vi "Check Chip Selection.vi"(6 "chip select":enum16{"1st chip", "2nd chip"}(ring), 8 "error in (no error)":errorcluster, 11 "cluster of private data in":T1={"FPGA VI Reference"=refnum, "device index"=0, "screen size"=enum."8x1", "font size"=enum."5x8", "auto wrap"=FALSE, "alignment"=enum."None", "number of line"=enum."2 lines", "shift 0"=0, "entry mode 0"=enum."increment & no shift", "shift 1"=0, "entry mode 1"=enum."increment & no shift"}) -> (0 "error out":errorcluster, 3 "cluster of private data out":T1={"FPGA VI Reference"=refnum, "device index"=0, "screen size"=enum."8x1", "font size"=enum."5x8", "auto wrap"=FALSE, "alignment"=enum."None", "number of line"=enum."2 lines", "shift 0"=0, "entry mode 0"=enum."increment & no shift", "shift 1"=0, "entry mode 1"=enum."increment & no shift"})   [LabVIEW 2017, in "HD44780.lvclass"]
uses:
  HD44780.lvclass
  Common/HD44780 Common.lvlib
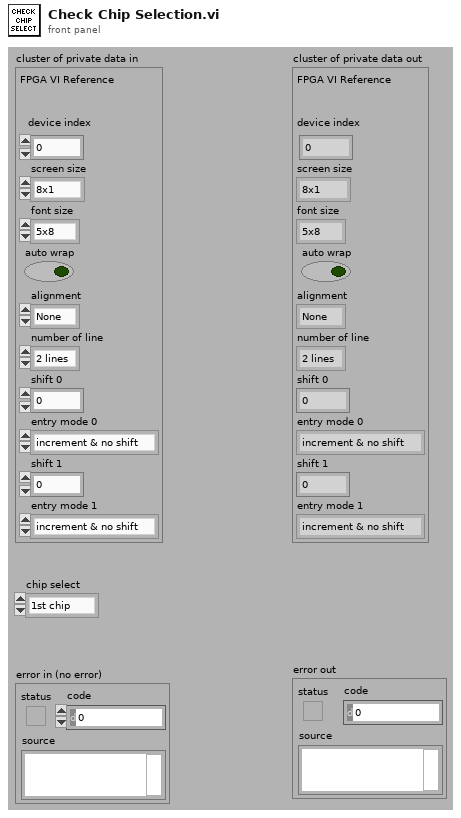
[diagram p1: front panel]
types:
  T1 = cluster{"FPGA VI Reference":refnum<k20>, "device index":i8, "screen size":enum8{"8x1", "8x2", "12x4", "16x1", "16x2", "16x4", "20x1", "20x2", "20x4", "24x1", "24x2", "40x2", "40x4"}, "font size":enum8{"5x8", "5x10"}, "auto wrap":bool, "alignment":enum16{"None", "Left", "Center", "Right"}, "number of line":enum8{"1 line", "2 lines"}, "shift 0":i8, "entry mode 0":enum8{"increment & no shift", "increment & shift", "decrement & no shift", "decrement & shift"}, "shift 1":i8, "entry mode 1":enum8{"increment & no shift", "increment & shift", "decrement & no shift", "decrement & shift"}}
  T2 = enum8{"8x1", "8x2", "12x4", "16x1", "16x2", "16x4", "20x1", "20x2", "20x4", "24x1", "24x2", "40x2", "40x4"}
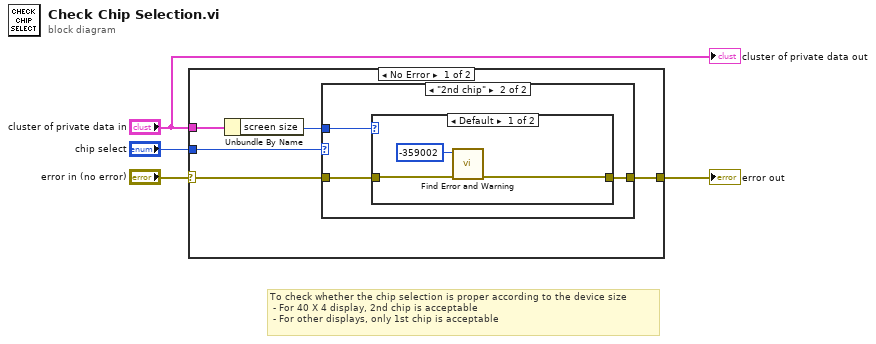
[diagram p0: block diagram]
diagram:
  # "To check whether the chip selection is proper according to the device size\n - For 40 X 4 display, 2nd chip is acceptable\n - For other displays, only 1st chip is acceptable"
  n1 = case shown="No Error" "error in (no error)" {
    selector: "error in (no error)" -> [w5 w18]
    tunnel: [w9 w18] -> w4
    tunnel: "chip select" -> [w8 _]
    tunnel: "cluster of private data in" -> [w6 _]
    frame No Error {
      n2 = Unbundle By Name(w6) -> ("screen size"=w7:T2)
      n3 = case shown="\"2nd chip\"" w8 {
        tunnel: [w10 w13] -> w9
        tunnel: w7 -> [_ w12]
        tunnel: w5 -> [w10 w11]
        frame "1st chip", Default {
        }
        frame "2nd chip" {
          n4 = case shown="Default" w12 {
            tunnel: [w16 w17] -> w13
            tunnel: w11 -> [w14 w17]
            frame Default {
              n5 = call "Find Error and Warning.vi"("error in (no error)"=w14, "error code"=-359002) -> ("error out"=w16:errorcluster)  [unwired: 9 in]
            }
            frame "40x4" {
            }
          }
        }
      }
    }
    frame Error {
    }
  }
  "error out" <- w4
  "cluster of private data out" <- "cluster of private data in"
